vi "Init Hail.vi"(8 "error in (no error)":errorcluster, 10 "Start Player":cluster{"Row":i32, "Column":i32}, 11 "Hail in":refnum<class "Hail.lvclass">) -> (0 "error out":errorcluster, 3 "Hail out":refnum<class "Hail.lvclass">)   [LabVIEW 2015, in "Hail.lvclass"]
uses:
  Hail.lvclass
  Group Cluster.ctl
  Mode Enum.ctl
  Board Cluster.ctl
  Hail.lvclass/Hail.ctl
  SubVIs/Read-Only Globals.vi
  SubVIs/Globals (private).vi
  Square/Square.lvclass
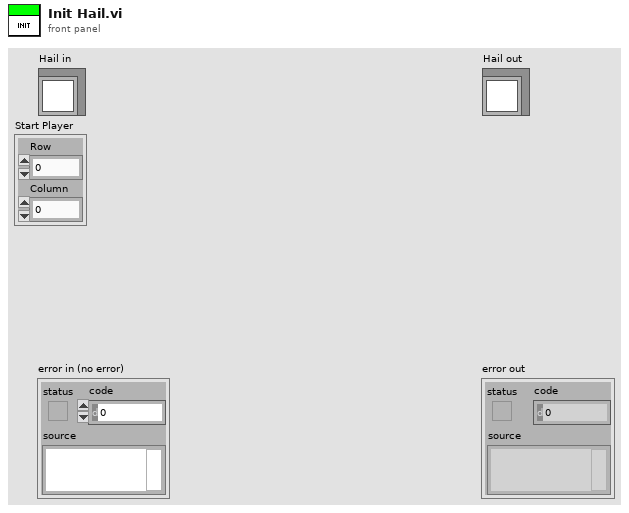
[diagram p1: front panel]
types:
  T1 = typedef "Hail.lvclass/Board Cluster.ctl" = cluster{"Group[][]":i32[][], "Center":cluster{"Col":i32, "Row":i32}, "Spread Dist":i32, "Radius Idx":i32, "Circum Idx":i32, "Attractor[][]":i32[][]}
  T2 = typedef "Hail.lvclass/Mode Enum.ctl" = enum16{"Grow(1)", "Grow(2)", "Grow(4)", "Grow(8)", "Divide", "Farewell", "Move"}
  T3 = typedef "Hail.lvclass/Group Cluster.ctl" = cluster{"Mode":T2, "Move Amt":i32, "Group Cnt":i32, "Temp":u32, "Round":i32}
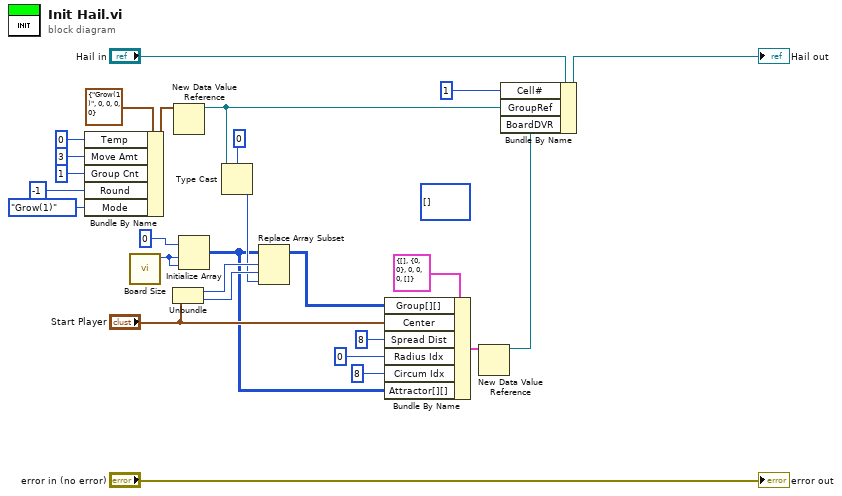
[diagram p0: block diagram]
diagram:
  (unwired) i32[][] [] ("Group[][]")
  n1 = Bundle By Name(cluster=T3 {"Mode"=enum."Grow(1)", "Move Amt"=0, "Group Cnt"=0, "Temp"=0, "Round"=0} ("Group Cluster"), "Temp"=u32 0, "Move Amt"=3, "Group Cnt"=1, "Round"=-1, "Mode"=Mode_Enum."Grow(1)") -> (w15:T3)
  n2 = call "Board Size.vi"() -> ("Board Size"=w17:i32)  [unwired: 11 in]
  n3 = Unbundle("Start Player") -> ("Row"=w7:i32, "Column"=w6:i32)
  n4 = New Data Value Reference(data value=w15) -> (data value reference=w4:refnum<data-value>)  [unwired: 1 in, 1 out]
  n5 = Initialize Array(0, w17, w17) -> (w1:i32[][])
  n6 = Type Cast(type=0, x=w4) -> (*(type *) &x=w3:i32)
  n7 = Replace Array Subset(array=w1, new element=w3, index (row)=w7, index (col)=w6) -> (w5:i32[][])
  n8 = Bundle By Name(cluster=T1 {"Group[][]"=[], "Center"={"Col"=0, "Row"=0}, "Spread Dist"=0, "Radius Idx"=0, "Circum Idx"=0, "Attractor[][]"=[]} ("Board"), "Group[][]"=w5, "Center"="Start Player", "Spread Dist"=8, "Radius Idx"=0, "Circum Idx"=8 ("Spread Dist"), "Attractor[][]"=w1) -> (w13:T1)
  n9 = New Data Value Reference(data value=w13) -> (data value reference=w12:refnum<data-value>)  [unwired: 1 in, 1 out]
  n10 = Bundle By Name(cluster="Hail in", "Cell#"=i8 1, "GroupRef"=w4, "BoardDVR"=w12) -> (→"Hail out":refnum<class "Hail.lvclass">)
  "error out" <- "error in (no error)"
